vi "Configure Output.vi"(0 "VISA resource name":refnum<visa-resource-name>, 5 "Output Mode (0: OFF)":u16(ring) items=["OFF", "CALSQ", "PF", "TRIG", "LEVEL", "ENABLED", "PULSE"], 7 "Level (1 V)":dbl=1.0, 9 "Rate (1 kHz)":dbl=1000.0, 11 "error in (no error)":errorcluster) -> (4 "VISA resource name out":refnum<visa-resource-name>, 15 "error out":errorcluster)   [LabVIEW 2015, in "LeCroy Wave Series.lvlib"]
doc: "Configures the type of signal put out through the instrument front panel’s CAL BNC connector."
uses:
  <instrlib>/LeCroy Wave Series/LeCroy Wave Series.lvlib
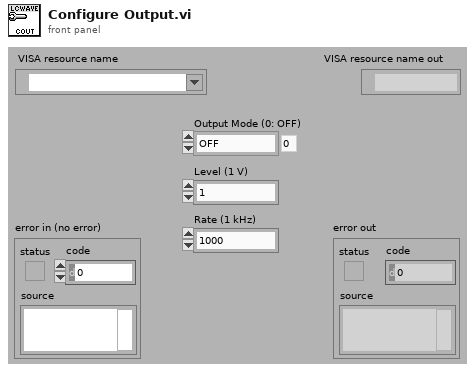
[diagram p1: front panel]
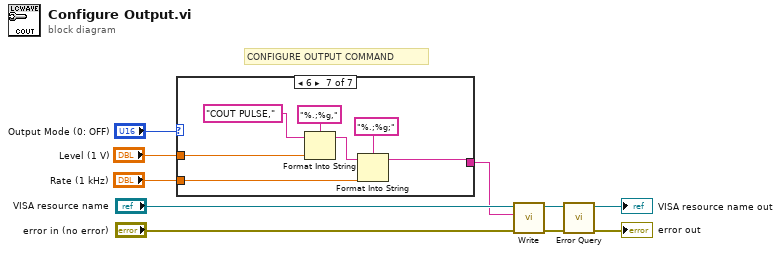
[diagram p0: block diagram]
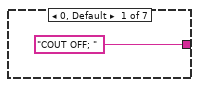
[diagram p2: hidden frame]
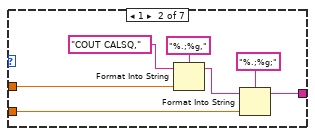
[diagram p3: hidden frame]
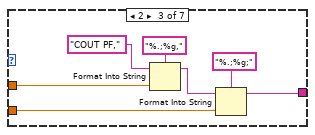
[diagram p4: hidden frame]
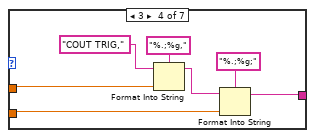
[diagram p5: hidden frame]
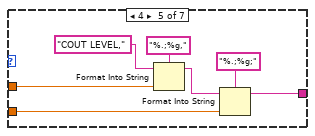
[diagram p6: hidden frame]
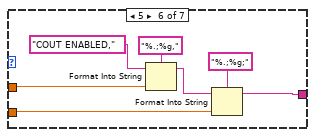
[diagram p7: hidden frame]
diagram:
  # "CONFIGURE OUTPUT COMMAND"
  n1 = case shown="6" "Output Mode (0: OFF)" {
    tunnel: "Level (1 V)" -> [_ w18 w21 w28 w35 w42 w51]
    tunnel: "Rate (1 kHz)" -> [_ w17 w20 w27 w34 w41 w49]
    tunnel: ["COUT OFF; " ("format string") w12 w19 w26 w33 w40 w47] -> w1
    frame 0, Default {
    }
    frame 1 {
      n2 = Format Into String(format string="%.;%g,", initial string="COUT CALSQ," ("format string"), w18) -> (resulting string=w14:string)  [unwired: 1 in, 1 out]
      n3 = Format Into String(format string="%.;%g;", initial string=w14, w17) -> (resulting string=w12:string)  [unwired: 1 in, 1 out]
    }
    frame 2 {
      n4 = Format Into String(format string="%.;%g,", initial string="COUT PF," ("format string"), w21) -> (resulting string=w23:string)  [unwired: 1 in, 1 out]
      n5 = Format Into String(format string="%.;%g;", initial string=w23, w20) -> (resulting string=w19:string)  [unwired: 1 in, 1 out]
    }
    frame 3 {
      n6 = Format Into String(format string="%.;%g,", initial string="COUT TRIG," ("format string"), w28) -> (resulting string=w30:string)  [unwired: 1 in, 1 out]
      n7 = Format Into String(format string="%.;%g;", initial string=w30, w27) -> (resulting string=w26:string)  [unwired: 1 in, 1 out]
    }
    frame 4 {
      n8 = Format Into String(format string="%.;%g,", initial string="COUT LEVEL," ("format string"), w35) -> (resulting string=w37:string)  [unwired: 1 in, 1 out]
      n9 = Format Into String(format string="%.;%g;", initial string=w37, w34) -> (resulting string=w33:string)  [unwired: 1 in, 1 out]
    }
    frame 5 {
      n10 = Format Into String(format string="%.;%g,", initial string="COUT ENABLED," ("format string"), w42) -> (resulting string=w44:string)  [unwired: 1 in, 1 out]
      n11 = Format Into String(format string="%.;%g;", initial string=w44, w41) -> (resulting string=w40:string)  [unwired: 1 in, 1 out]
    }
    frame 6 {
      n12 = Format Into String(format string="%.;%g,", initial string="COUT PULSE," ("format string"), w51) -> (resulting string=w48:string)  [unwired: 1 in, 1 out]
      n13 = Format Into String(format string="%.;%g;", initial string=w48, w49) -> (resulting string=w47:string)  [unwired: 1 in, 1 out]
    }
  }
  n14 = call <instrlib>:"Write.vi"("error in (no error)"="error in (no error)", "Write Buffer"=w1, "VISA resource name"="VISA resource name") -> ("error out"=w5:errorcluster, "VISA resource name out"=w6:refnum<visa-resource-name>)  [unwired: 6 in, 1 out]
  n15 = call <instrlib>:"Error Query.vi"("error in (no error)"=w5, "VISA resource name"=w6) -> ("error out"=→"error out":errorcluster, "VISA resource name out"=→"VISA resource name out":refnum<visa-resource-name>)  [unwired: 6 in, 2 out]
